vi "Read status.vi"(8 "error in (no error)":errorcluster, 11 "PV in":refnum<class "PV.lvclass">) -> (0 "error out":errorcluster, 2 "Status":i32, 3 "PV out":refnum<class "PV.lvclass">)   [LabVIEW 2012, in "CS++ProcessVariables.lvlib" / "PV.lvclass"]
doc: "Read Status."
uses:
  PV.lvclass
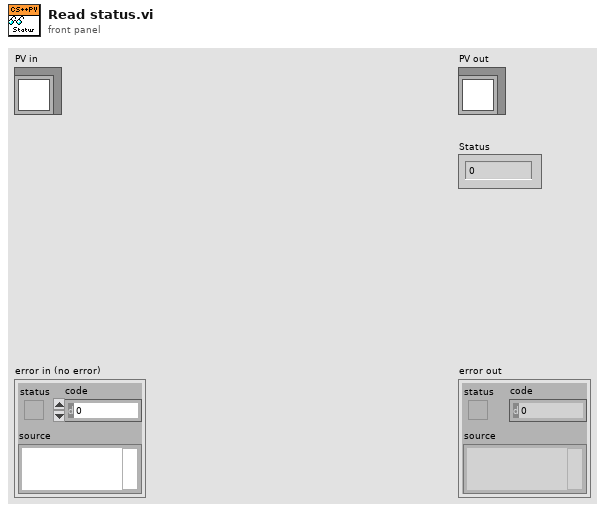
[diagram p1: front panel]
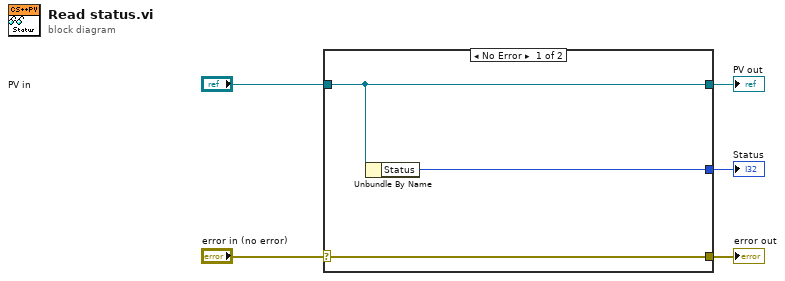
[diagram p0: block diagram]
diagram:
  n1 = case shown="No Error" "error in (no error)" {
    selector: "error in (no error)" -> [w8 w9]
    tunnel: [w8 w9] -> w4
    tunnel: [w7 w10] -> w2
    tunnel: "PV in" -> [w7 w10]
    tunnel: [w6 _] -> w1
    frame No Error {
      n2 = Unbundle By Name(w7) -> ("Status"=w6:u32)
    }
    frame Error {
    }
  }
  "error out" <- w4
  "PV out" <- w2
  "Status" <- w1
